vi "Set Environment Variable.vi"(7 "Target (Process)":T1 items=["Process", "User", "Machine"], 8 "Error In":errorcluster, 10 "Value":string, 11 "Name":string) -> (0 "Error Out":errorcluster)   [LabVIEW 2023, in "SLL Environment Variable.lvlib"]
doc: "Set <B>Value</B> to the environment variable in the target environment."
uses:
  SLL Environment Variable.lvlib
  _Typedef/Target Environment Enum.ctl
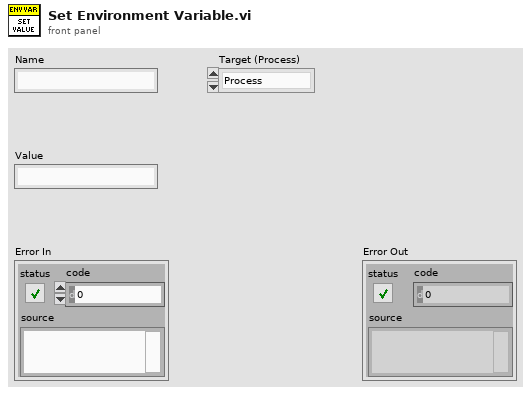
[diagram p1: front panel]
types:
  T1 = typedef "SLL Environment Variable.lvlib/Target Environment Enum.ctl" = i32
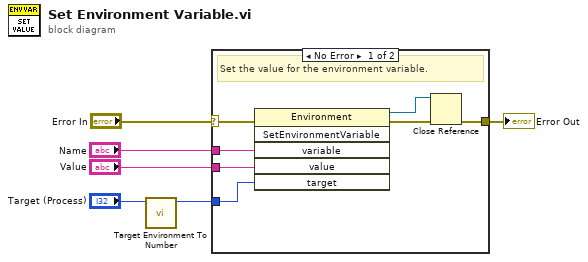
[diagram p0: block diagram]
diagram:
  n1 = call "Target Environment To Number.vi"("Target (Process)"="Target (Process)") -> ("Number"=w1:i32)  [unwired: 10 in]
  n2 = case shown="No Error" "Error In" {
    selector: "Error In" -> [w13 w14]
    tunnel: "Name" -> [w12 _]
    tunnel: [w10 w14] -> w4
    tunnel: "Value" -> [w8 _]
    tunnel: w1 -> [w7 _]
    frame No Error {
      # "Set the value for the environment variable."
      n3 = invoke class="Environment" method="SetEnvironmentVariable"(error in=w13, "variable"=w12, "value"=w8, "target"=w7) -> (reference out=w9:refnum<k24>, error out=w11:errorcluster)  [unwired: 2 in, 4 out]
      n4 = Close Reference(reference=w9, error in (no error)=w11) -> (error out=w10:errorcluster)
    }
    frame Error {
    }
  }
  "Error Out" <- w4
